vi "VI Server_GetControlClassNameAndTypeFromGenericRef.vi"(8 "error in (no error)":errorcluster, 9 "Control Reference":refnum<vi>) -> (0 "error out":errorcluster, 1 "ClassName":string, 2 "ControlType":T1, 5 "ControlLabel":string)   [LabVIEW 2020, in "VI Server Toolkit LV2013.lvlib"]
doc: "Returns control class name and its type (digital, Boolean, etc.)\nRequires \"generic\" control's reference input."
uses:
  VI Server Toolkit LV2013.lvlib
  VI Server_TypeDefs/VI Server_DataType.ctl
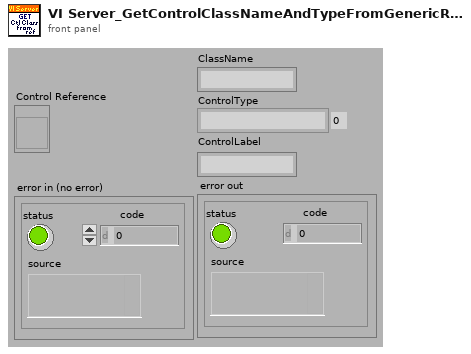
[diagram p1: front panel]
types:
  T1 = typedef "VI Server Toolkit LV2013.lvlib/VI Server_DataType.ctl" = enum16{"", "Digital [Dbl]", "Digital [Sgl]", "Digital [I32]", "Digital [I16]", "Digital [I8]", "Digital [U32]", "Digital [U16]", "Digital [U8]", "Boolean", "Slide [Dbl]", "Slide [Sgl]", "Slide [I32]", "Slide [I16]", "Slide [I8]", "Slide [U32]", "Slide [U16]", "Slide [U8]", "Enumerated", "Path", "VISA Resource Name", "Text Ring", "String", "TabControl", "Knob [U8]", "Knob [U16]", "Knob [U32]", "Knob [I8]", "Knob [I16]", "Knob [I32]", "Knob [SGL]", "Knob [DBL]"}
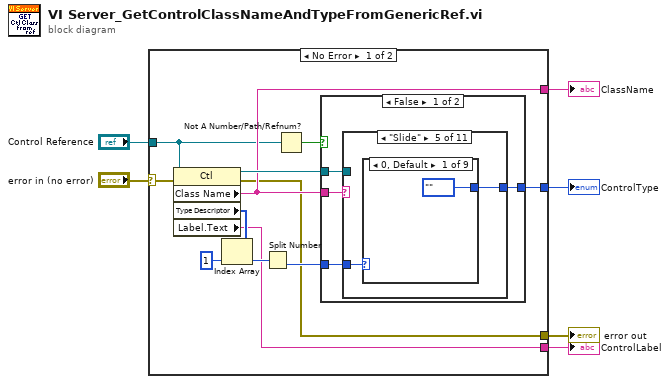
[diagram p0: block diagram]
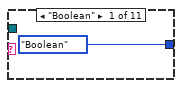
[diagram p2: hidden frame]
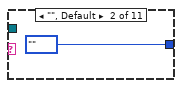
[diagram p3: hidden frame]
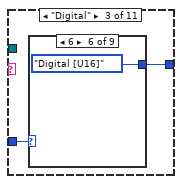
[diagram p4: hidden frame]
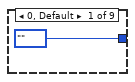
[diagram p5: hidden frame]
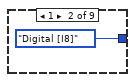
[diagram p6: hidden frame]
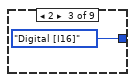
[diagram p7: hidden frame]
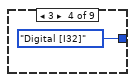
[diagram p8: hidden frame]
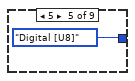
[diagram p9: hidden frame]
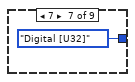
[diagram p10: hidden frame]
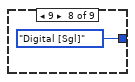
[diagram p11: hidden frame]
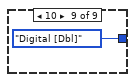
[diagram p12: hidden frame]
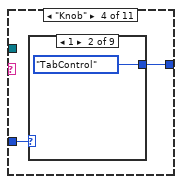
[diagram p13: hidden frame]
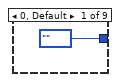
[diagram p14: hidden frame]
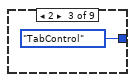
[diagram p15: hidden frame]
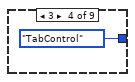
[diagram p16: hidden frame]
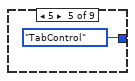
[diagram p17: hidden frame]
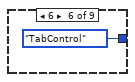
[diagram p18: hidden frame]
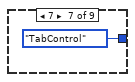
[diagram p19: hidden frame]
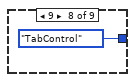
[diagram p20: hidden frame]
diagram:
  n1 = case shown="No Error" "error in (no error)" {
    selector: "error in (no error)" -> [w10 w66]
    tunnel: [w7 w66] -> w6
    tunnel: [w12 VI_Server_DataType."" ("ControlType 2")] -> w4
    tunnel: [w11 _] -> w3
    tunnel: "Control Reference" -> [w9 _]
    tunnel: [w8 _] -> w1
    frame No Error {
      n2 = property class="Ctl"(reference=w9, error in=w10) -> (reference out=w14:refnum<vi>, error out=w7:errorcluster, "Class Name"=w11:string, "Type Descriptor"=w16:i16[], "Label.Text"=w8:string)
      n3 = Index Array(array=w16, index=1) -> (element=w17:i16)
      n4 = Split Number(x=w17) -> (lo(x)=w15:u8)  [unwired: 1 out]
      n5 = Not A Number/Path/Refnum?(number/path/refnum=w9) -> (NaN/Path/Refnum?=w13:bool)
      n6 = case shown="False" w13 {
        tunnel: w11 -> [w22 _]
        tunnel: w15 -> [w21 _]
        tunnel: w14 -> [w20 _]
        tunnel: [w19 VI_Server_DataType."" ("ControlType 2")] -> w12
        frame False {
          n7 = case shown="\"Slide\"" w22 {
            tunnel: w21 -> [_ _ w26 w37 w48 _ _ _ _ _ _]
            tunnel: w20 -> [_ _ _ _ _ _ _ _ _ _ _]
            tunnel: [VI_Server_DataType."Boolean" ("ControlType 2") VI_Server_DataType."" ("ControlType 2") w25 w36 w47 VI_Server_DataType."Enumerated" ("ControlType 2") VI_Server_DataType."Path" ("ControlType 2") VI_Server_DataType."VISA Resource Name" ("ControlType 2") VI_Server_DataType."Text Ring" ("ControlType 2") VI_Server_DataType."String" ("ControlType 2") VI_Server_DataType."TabControl" ("ControlType 2")] -> w19
            frame "Boolean" {
            }
            frame "", Default {
            }
            frame "Digital" {
              n8 = case shown="6" w26 {
                tunnel: [VI_Server_DataType."" ("ControlType 2") VI_Server_DataType."Digital [I8]" ("ControlType 2") VI_Server_DataType."Digital [I16]" ("ControlType 2") VI_Server_DataType."Digital [I32]" ("ControlType 2") VI_Server_DataType."Digital [U8]" ("ControlType 2") VI_Server_DataType."Digital [U16]" ("ControlType 2") VI_Server_DataType."Digital [U32]" ("ControlType 2") VI_Server_DataType."Digital [Sgl]" ("ControlType 2") VI_Server_DataType."Digital [Dbl]" ("ControlType 2")] -> w25
                frame 0, Default {
                }
                frame 1 {
                }
                frame 2 {
                }
                frame 3 {
                }
                frame 5 {
                }
                frame 6 {
                }
                frame 7 {
                }
                frame 9 {
                }
                frame 10 {
                }
              }
            }
            frame "Knob" {
              n9 = case shown="1" w37 {
                tunnel: [VI_Server_DataType."" ("ControlType 2") VI_Server_DataType."TabControl" ("ControlType 2") VI_Server_DataType."TabControl" ("ControlType 2") VI_Server_DataType."TabControl" ("ControlType 2") VI_Server_DataType."TabControl" ("ControlType 2") VI_Server_DataType."TabControl" ("ControlType 2") VI_Server_DataType."TabControl" ("ControlType 2") VI_Server_DataType."TabControl" ("ControlType 2") VI_Server_DataType."TabControl" ("ControlType 2")] -> w36
                frame 0, Default {
                }
                frame 1 {
                }
                frame 2 {
                }
                frame 3 {
                }
                frame 5 {
                }
                frame 6 {
                }
                frame 7 {
                }
                frame 9 {
                }
                frame 10 {
                }
              }
            }
            frame "Slide" {
              n10 = case shown="0, Default" w48 {
                tunnel: [VI_Server_DataType."" ("ControlType 2") VI_Server_DataType."Slide [I8]" ("ControlType 2") VI_Server_DataType."Slide [I16]" ("ControlType 2") VI_Server_DataType."Slide [I32]" ("ControlType 2") VI_Server_DataType."Slide [U8]" ("ControlType 2") VI_Server_DataType."Slide [U16]" ("ControlType 2") VI_Server_DataType."Slide [U32]" ("ControlType 2") VI_Server_DataType."Slide [Sgl]" ("ControlType 2") VI_Server_DataType."Slide [Dbl]" ("ControlType 2")] -> w47
                frame 0, Default {
                }
                frame 1 {
                }
                frame 2 {
                }
                frame 3 {
                }
                frame 5 {
                }
                frame 6 {
                }
                frame 7 {
                }
                frame 9 {
                }
                frame 10 {
                }
              }
            }
            frame "Enum" {
            }
            frame "Path" {
            }
            frame "VISAResourceName" {
            }
            frame "Ring" {
            }
            frame "String" {
            }
            frame "TabControl" {
            }
          }
        }
        frame True {
          (unwired) ""
        }
      }
    }
    frame Error {
    }
  }
  "error out" <- w6
  "ControlType" <- w4
  "ClassName" <- w3
  "ControlLabel" <- w1
